vi "Read 1 binned horiz.vi"(0 "Nmb of  img row":i32=300, 1 "sensitivity":dbl=1.0, 2 "data":dbl[](array[numeric])=[12276.0, 13132.0, 13286.0, 13664.0, 13368.0, 13938.0, 12728.0, 13051.0, 14692.0, 14393.0, 14369.0, 14214.0, 13813.0, 14019.0, 13792.0, 14074.0, 13638.0, 14005.0, 14097.0, 14201.0, 13510.0, 13553.0, 13639.0, 13373.0, 13618.0, 13543.0, 12957.0, 13480.0, 13524.0, 13547.0, 13530.0, 12880.0, 13534.0, 13764.0, 13395.0, 13340.0, 13031.0, 13400.0, 13264.0, 12351.0, 12776.0, 12590.0, 13115.0, 12455.0, 12730.0, 12069.0, 12295.0, 12526.0, 11885.0, 12306.0, 11400.0, 11819.0, 11633.0, 11699.0, 11383.0, 11286.0, 10687.0, 11336.0, 11139.0, 11061.0, 10970.0, 11173.0, 10301.0, 10884.0, 10507.0, 10762.0, 10316.0, 10198.0, 10378.0, 10286.0, 10597.0, 9988.0, 9757.0, 10236.0, 10107.0, 9669.0, 9647.0, 9879.0, 9491.0, 9436.0, 9804.0, 9619.0, 9596.0, 9884.0, 9894.0, 9050.0, 9035.0, 9463.0, 9079.0, 9190.0, 9159.0, 9163.0, 9499.0, 9468.0, 8895.0, 9148.0, 8875.0, 9351.0, 8978.0, 8600.0, 8447.0, 8981.0, 8905.0, 8318.0, 8773.0, 8796.0, 8339.0, 8345.0, 8314.0, 8365.0, 8654.0, 8171.0, 8417.0, 8169.0, 8625.0, 8569.0, 8231.0, 8509.0, 8338.0, 8334.0, 7922.0, 8058.0, 8318.0, 8263.0, 7984.0, 8210.0, 8218.0, 8265.0, 8390.0, 8217.0, 7726.0, 8073.0, 8113.0, 7884.0, 7563.0, 8068.0, 8215.0, 7885.0, 8043.0, 7827.0, 7685.0, 7631.0, 7792.0, 8733.0, 8167.0, 7931.0, 7764.0, 8282.0, 7973.0, 8214.0, 7596.0, 7719.0, 8173.0, 7901.0, 7975.0, 7934.0, 7774.0, 8203.0, 8416.0, 8202.0, 8166.0, 8353.0, 8369.0, 8414.0, 8184.0, 7953.0, 8008.0, 8602.0, 8295.0, 8616.0, 7993.0, 8121.0, 8311.0], 3 "BG":dbl[](array[numeric])=[12276.0, 13132.0, 13286.0, 13664.0, 13368.0, 13938.0, 12728.0, 13051.0, 14692.0, 14393.0, 14369.0, 14214.0, 13813.0, 14019.0, 13792.0, 14074.0, 13638.0, 14005.0, 14097.0, 14201.0, 13510.0, 13553.0, 13639.0, 13373.0, 13618.0, 13543.0, 12957.0, 13480.0, 13524.0, 13547.0, 13530.0, 12880.0, 13534.0, 13764.0, 13395.0, 13340.0, 13031.0, 13400.0, 13264.0, 12351.0, 12776.0, 12590.0, 13115.0, 12455.0, 12730.0, 12069.0, 12295.0, 12526.0, 11885.0, 12306.0, 11400.0, 11819.0, 11633.0, 11699.0, 11383.0, 11286.0, 10687.0, 11336.0, 11139.0, 11061.0, 10970.0, 11173.0, 10301.0, 10884.0, 10507.0, 10762.0, 10316.0, 10198.0, 10378.0, 10286.0, 10597.0, 9988.0, 9757.0, 10236.0, 10107.0, 9669.0, 9647.0, 9879.0, 9491.0, 9436.0, 9804.0, 9619.0, 9596.0, 9884.0, 9894.0, 9050.0, 9035.0, 9463.0, 9079.0, 9190.0, 9159.0, 9163.0, 9499.0, 9468.0, 8895.0, 9148.0, 8875.0, 9351.0, 8978.0, 8600.0, 8447.0, 8981.0, 8905.0, 8318.0, 8773.0, 8796.0, 8339.0, 8345.0, 8314.0, 8365.0, 8654.0, 8171.0, 8417.0, 8169.0, 8625.0, 8569.0, 8231.0, 8509.0, 8338.0, 8334.0, 7922.0, 8058.0, 8318.0, 8263.0, 7984.0, 8210.0, 8218.0, 8265.0, 8390.0, 8217.0, 7726.0, 8073.0, 8113.0, 7884.0, 7563.0, 8068.0, 8215.0, 7885.0, 8043.0, 7827.0, 7685.0, 7631.0, 7792.0, 8733.0, 8167.0, 7931.0, 7764.0, 8282.0, 7973.0, 8214.0, 7596.0, 7719.0, 8173.0, 7901.0, 7975.0, 7934.0, 7774.0, 8203.0, 8416.0, 8202.0, 8166.0, 8353.0, 8369.0, 8414.0, 8184.0, 7953.0, 8008.0, 8602.0, 8295.0, 8616.0, 7993.0, 8121.0, 8311.0], 4 "vignette":dbl[](array[numeric])) -> (5 "Output":dbl[](array[numeric]))   [LabVIEW 2013]
uses:
  <vilib>/Analysis/2dsp.llb/Decimate (single shot, DBL).vi
  <vilib>/Analysis/NI_AALPro.lvlib
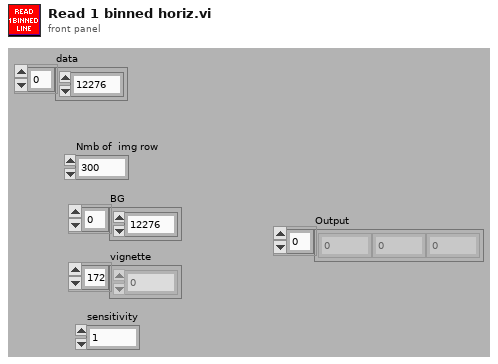
[diagram p1: front panel]
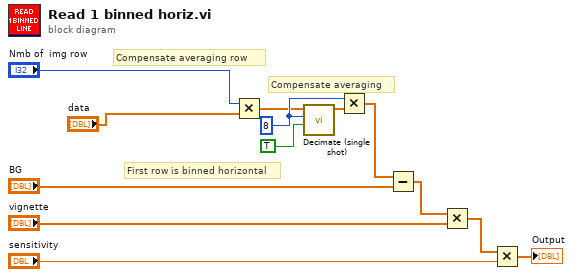
[diagram p0: block diagram]
diagram:
  w10 = 8 ("decimating factor")
  # "Compensate averaging"
  # "Compensate averaging row"
  # "First row is binned horizontal"
  n1 = Multiply(x="Nmb of  img row", y="data") -> (x*y=w9:dbl[])
  n2 = call-poly <vilib>:"Decimate (single shot).vi"("averaging"=TRUE, "decimating factor"=w10, "X"=w9) -> ("Decimated Array"=w11:dbl[])  [unwired: 7 in, 1 out]
  n3 = Multiply(x=w10, y=w11) -> (x*y=w5:dbl[])
  n4 = Subtract(x=w5, y="BG") -> (x-y=w6:dbl[])
  n5 = Multiply(x=w6, y="vignette") -> (x*y=w3:dbl[])
  n6 = Multiply(x=w3, y="sensitivity") -> (x*y=→"Output":dbl[])
